vi "ziModRead.vi"(8 "error in":errorcluster, 11 "ziModHandle In":T1 {"ModHandle" format="0x%08x"; "Conn" format="0x%08x"}) -> (0 "error out":errorcluster, 3 "ziModHandle Out":T1 {"ModHandle" format="0x%08x"; "Conn" format="0x%08x"})   [LabVIEW 2018, in "Zurich Instruments LabOne.lvlib"]
doc: "ModRead polls the all data no matter if the module is finished from the device. Finished Data and partly processed data are returned and deleted from the device. \n\nUse ziGetNextNode in order to access all the availible data."
uses:
  Zurich Instruments LabOne.lvlib
  <instrlib>/Zurich Instruments LabOne/Private/ziLV64.framework
  ziTypeModHandle.ctl
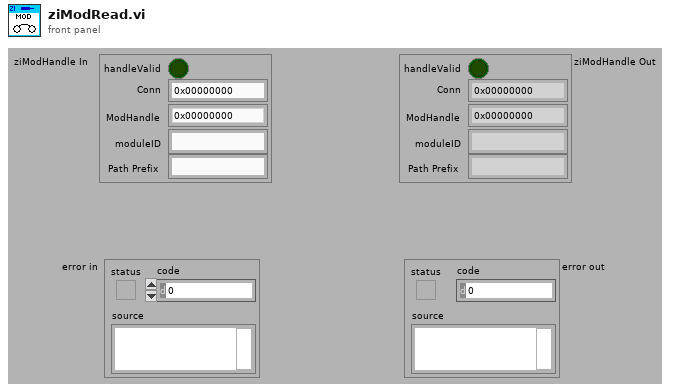
[diagram p1: front panel]
types:
  T1 = typedef "Zurich Instruments LabOne.lvlib/ziTypeModHandle.ctl" = cluster{"handleValid":bool, "Conn":u64, "ModHandle":u64, "moduleID":string, "Path Prefix":string}
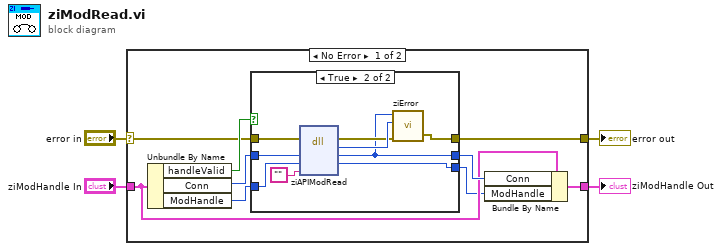
[diagram p0: block diagram]
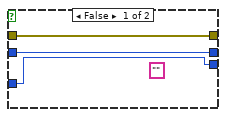
[diagram p2: hidden frame]
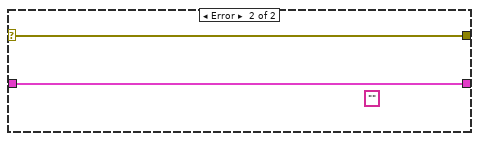
[diagram p3: hidden frame]
diagram:
  n1 = case shown="No Error" "error in" {
    selector: "error in" -> [w8 w27]
    tunnel: [w13 w27] -> w4
    tunnel: [w9 w26] -> w1
    tunnel: "ziModHandle In" -> [w7 w26]
    frame No Error {
      n2 = Unbundle By Name(w7) -> ("handleValid"=w12:bool, "Conn"=w11:u64, "ModHandle"=w6:u64)
      n3 = case shown="True" w12 {
        tunnel: w8 -> [w16 w25]
        tunnel: w11 -> [w15 w24]
        tunnel: [w15 w17] -> w10
        tunnel: [w16 w18] -> w13
        tunnel: w6 -> [w14 w23]
        tunnel: [w14 w19] -> w5
        frame False {
          (unwired) "" ("Path")
        }
        frame True {
          n4 = dll-call lib="Applications/National Instruments/LabVIEW 2019 64-bit/instr.lib/Zurich Instruments LabOne/Private/ziLV*.*" fn="ziAPIModRead"(error in=w25, "Conn"=w24, "ModHandle"=w23, "Path"="") -> (error out=w21:errorcluster, "return type"=w22:u32, "Conn"=w17:u64, "ModHandle"=w19:u64)  [unwired: 3 in, 1 out]
          n5 = call "ziError.vi"("Conn"=w17, "ziErrorCode"=w22, "Error In"=w21) -> ("Error Out"=w18:errorcluster)  [unwired: 2 in, 1 out]
        }
      }
      n6 = Bundle By Name(cluster=w7, "Conn"=w10, "ModHandle"=w5) -> (w9:T1)
    }
    frame Error {
      (unwired) "" ("Path")
    }
  }
  "error out" <- w4
  "ziModHandle Out" <- w1
